vi "FlatToRichnidevice_grpc_Session.vi"(5 "OutputClusterType":T1, 11 "InputCluster":T2) -> (3 "OutputCluster":T1)   [LabVIEW 2021, in "NI Switch_client.lvlib"]
uses:
  NI Switch_client.lvlib
  nidevice_grpc_Session_Flat.ctl
  nidevice_grpc_Session.ctl
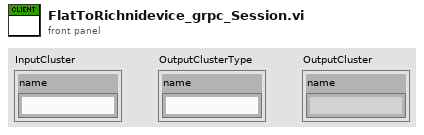
[diagram p1: front panel]
types:
  T1 = typedef "NI Switch_client.lvlib/nidevice_grpc_Session.ctl" = cluster{"name":string}
  T2 = typedef "NI Switch_client.lvlib/nidevice_grpc_Session_Flat.ctl" = cluster{"name":string}
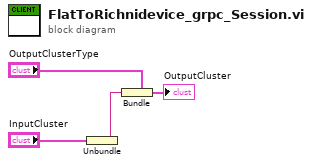
[diagram p0: block diagram]
diagram:
  n1 = Unbundle "Unbundle"("InputCluster") -> ("name"=w1:string)
  n2 = Bundle "Bundle"(cluster="OutputClusterType", "name"=w1) -> (→"OutputCluster":T1)
